vi "AddLabelsInMainGroup.vi"(0 "Engine In":refnum<k7>, 5 "SequenceFile In":refnum<k7>, 11 "Error In":errorcluster) -> (4 "Engine Out":refnum<k7>, 6 "SequenceFile Out":refnum<k7>, 15 "Error Out":errorcluster)   [LabVIEW 2021, in "Create Sequence.lvlib"]
doc: "Adds the required instruction steps on the 'MainGroup'"
uses:
  Create Sequence.lvlib
  TypeDef/StepProperties.ctl
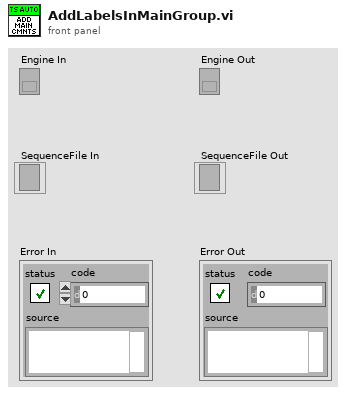
[diagram p1: front panel]
types:
  T1 = typedef "Create Sequence.lvlib/StepProperties.ctl" = cluster{"StepTypeName":string, "StepName":string, "Description":string, "Comment":string, "sequenceNameParam":string, "Step Group":i32, "Step Index":i32, "Expression":string}
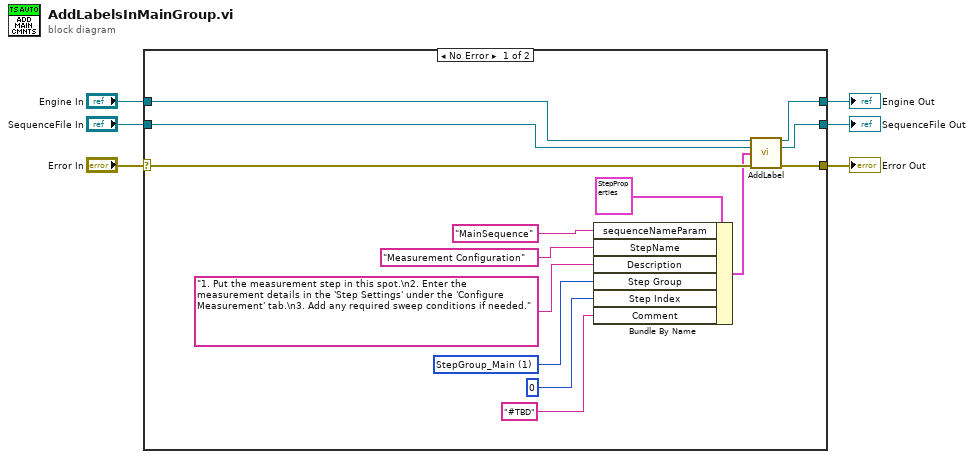
[diagram p0: block diagram]
diagram:
  n1 = case shown="No Error" "Error In" {
    selector: "Error In" -> [w20 w23]
    tunnel: "Engine In" -> [w16 w21]
    tunnel: "SequenceFile In" -> [w18 w22]
    tunnel: [w15 w21] -> w3
    tunnel: [w17 w22] -> w2
    tunnel: [w19 w23] -> w1
    frame No Error {
      w11 = 1 items=["StepGroup_Setup", "StepGroup_Main", "StepGroup_Cleanup"] ("Step Group")
      n2 = Bundle By Name(cluster=T1 {"StepTypeName"="", "StepName"="", "Description"="", "Comment"="", "sequenceNameParam"="MainSequence", "Step Group"=0, "Step Index"=3, "Expression"=""} ("StepProperties"), "sequenceNameParam"="MainSequence", "StepName"="Measurement Configuration" ("Step Name"), "Description"="1. Put the measurement step in this spot.\n2. Enter the measurement details in the 'Step Settings' under the 'Configure Measurement' tab.\n3. Add any required sweep conditions if needed.", "Step Group"=w11, "Step Index"=0, "Comment"="#TBD") -> (w9:T1)
      n3 = call "AddLabel.vi"("Engine In"=w16, "SequenceFile In"=w18, "StepProperties"=w9, "Error In"=w20) -> ("Engine Out"=w15:refnum<k7>, "SequenceFile Out"=w17:refnum<k7>, "Error Out"=w19:errorcluster)  [unwired: 9 in]
    }
    frame Error {
    }
  }
  "Error Out" <- w1
  "Engine Out" <- w3
  "SequenceFile Out" <- w2
